vi "test_BuildExternalDepSolutionWithVersion.vi"() -> (3 "Pass?":bool)   [LabVIEW 2019, in "Tests.SolutionBuilder.lvlib"]
uses:
  Tests.SolutionBuilder.lvlib
  SolutionBuilder/SolutionBuilder.lvclass
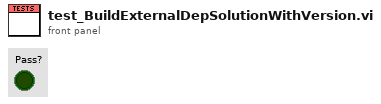
[diagram p1: front panel]
types:
  T1 = typedef "SolutionBuilder.lvlib/BuildManager.lvclass/GeneratedFile.ctl" = map{T2, set{string}}
  T2 = typedef "SolutionBuilder.lvlib/BuildManager.lvclass/BuildProjectInfo.ctl" = cluster{"Project path":string, "Build spec name":string, "Target":string}
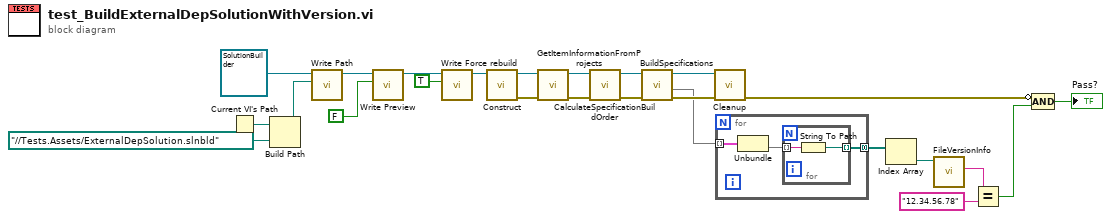
[diagram p0: block diagram]
diagram:
  n1 = Current VI's Path() -> (path=w23:path)
  n2 = Build Path(base path=w23, name or relative path=path "../../Tests.Assets/ExternalDepSolution.slnbld" ("Path")) -> (appended path=w21:path)
  n3 = call "Write Path.vi"("Path"=w21, "SolutionBuilder in"=refnum<class "SolutionBuilder.lvclass"> refnum) -> ("SolutionBuilder out"=w12:refnum<class "SolutionBuilder.lvclass">)  [unwired: 9 in]
  n4 = call "Write Preview.vi"("Preview?"=FALSE, "SolutionBuilder in"=w12) -> ("SolutionBuilder out"=w10:refnum<class "SolutionBuilder.lvclass">)  [unwired: 9 in]
  n5 = call "Write Force rebuild.vi"("Force rebuild"=TRUE, "SolutionBuilder in"=w10) -> ("SolutionBuilder out"=w9:refnum<class "SolutionBuilder.lvclass">)  [unwired: 9 in]
  n6 = call "Construct.vi"("SolutionBuilder in"=w9) -> ("error out"=w17:errorcluster, "SolutionBuilder out"=w20:refnum<class "SolutionBuilder.lvclass">)  [unwired: 9 in]
  n7 = call "GetItemInformationFromProjects.vi"("error in (no error)"=w17, "SolutionBuilder in"=w20) -> ("error out"=w16:errorcluster, "SolutionBuilder out"=w19:refnum<class "SolutionBuilder.lvclass">)  [unwired: 8 in]
  n8 = call "CalculateSpecificationBuildOrder.vi"("error in (no error)"=w16, "SolutionBuilder in"=w19) -> ("error out"=w15:errorcluster, "SolutionBuilder out"=w18:refnum<class "SolutionBuilder.lvclass">)  [unwired: 8 in]
  n9 = call "BuildSpecifications.vi"("error in (no error)"=w15, "SolutionBuilder in"=w18) -> ("error out"=w14:errorcluster, "Generated file"=w7:T1, "SolutionBuilder out"=w13:refnum<class "SolutionBuilder.lvclass">)  [unwired: 7 in]
  n10 = call "Cleanup.vi"("error in (no error)"=w14, "SolutionBuilder in"=w13) -> ("error out"=w6:errorcluster)  [unwired: 8 in, 1 out]
  n11 = for {
    tunnel: w7 -> [w28] mode=indexing
    tunnel: [w26] -> w5 mode=concatenating
    n12 = Unbundle(w28) -> ("Generated files"=w27:set{string})  [unwired: 1 out]
    n13 = for {
      tunnel: w27 -> [w30] mode=indexing
      tunnel: [w29] -> w26 mode=indexing
      n14 = String To Path(string=w30) -> (path=w29:path)
    }
  }
  n15 = Index Array(array=w5) -> (element=w4:path)  [unwired: 1 in]
  n16 = call <vilib>:"FileVersionInfo.vi"("Application Path in"=w4) -> ("File Version Info"=w3:string)  [unwired: 7 in, 3 out]
  n17 = Equal?(x=w3, y="12.34.56.78") -> (x = y?=w1:bool)
  n18 = Compound Arithmetic op=AND(invert w6, w1) -> (→"Pass?":bool)
